vi "ITC503 Set Values.vi"(1 "Set Heater":dbl min=0.0 max=100.0 step=0.1 format="%.1f", 2 "Set Channel":i16 min=0 max=100 step=1, 3 "ITC503 Settings":T1={"ITC503 Set Setpoint"=0.0, "ITC503 Set Auto Heater"=TRUE, "ITC503 Set Auto PID"=TRUE, "P"=0.0, "I"=0.0, "D"=0.0} {"D" min=0.0 max=100.0 step=0.1 format="%.1f"; "I" min=0.0 max=100.0 step=0.1 format="%.1f"; "P" min=0.0 max=100.0 step=0.1 format="%.1f"; "ITC503 Set Setpoint" min=-273.0 max=300000.0 step=0.1 format="%.1f"}, 4 "ITC Setup":T2={"Description"="", "IO Info"={"Address"={"Com Port"=1, "ISOBUS Address"=1, "GPIB Address"=24, "Communication"=enum."ISOBUS"}, "Version"=enum."ITC503", "Ch 1 dec places"=1, "Ch 2 dec places"=1, "Ch 3 dec places"=1, "Ch1 Name"="", "Ch2 Name"="", "Ch3 Name"=""}}) -> ()   [LabVIEW 2010]
uses:
  drivers/Oxford ITC/ITCAPPS.LLB/ITCSetup.ctl
  drivers/Oxford ITC/ITCSUBS.LLB/ITCIO.ctl
  drivers/Oxford ITC/BUSGEN.LLB/OxfordAddress.ctl
  drivers/Oxford ITC/ITCSUBS.LLB/ITCVersion.ctl
  TypeDefs/ITC503 Settings.ctl
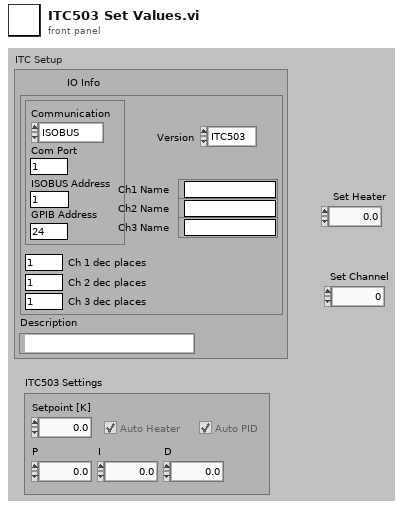
[diagram p1: front panel]
types:
  T1 = typedef "ITC503 Settings.ctl" = cluster{"ITC503 Set Setpoint":dbl, "ITC503 Set Auto Heater":bool, "ITC503 Set Auto PID":bool, "P":dbl, "I":dbl, "D":dbl}
  T2 = typedef "ITCSetup.ctl" = cluster{"Description":string, "IO Info":T3}
  T3 = typedef "ITCIO.ctl" = cluster{"Address":T4, "Version":T5, "Ch 1 dec places":i16, "Ch 2 dec places":i16, "Ch 3 dec places":i16, "Ch1 Name":string, "Ch2 Name":string, "Ch3 Name":string}
  T4 = typedef "OxfordAddress.ctl" = cluster{"Com Port":i32, "ISOBUS Address":i32, "GPIB Address":i16, "Communication":enum16{"RS232", "ISOBUS", "GPIB", "Gateway"}}
  T5 = typedef "ITCVersion.ctl" = enum16{"ITC502", "ITC503", "ITC601"}
  T6 = typedef "ITC503 Current Values.ctl" = cluster{"ITC503 Heater":dbl, "ITC503 Temperature":dbl, "ITC503 P":dbl, "ITC503 I":dbl, "ITC503 D":dbl, "ITC503 Setpoint":dbl, "ITC503 Gradient":dbl, "ITC503 Heater Auto":bool, "ITC503 PID Auto":bool}
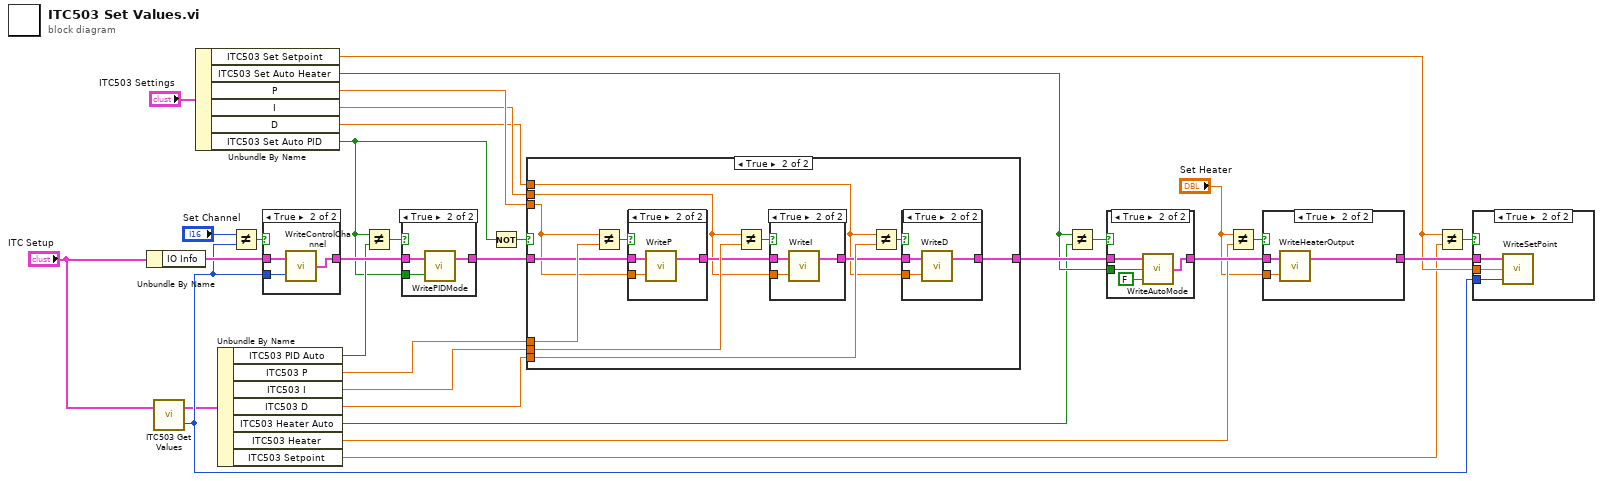
[diagram p0: block diagram]
diagram:
  n1 = Unbundle By Name("ITC Setup") -> ("IO Info"=w27:T3)
  n2 = call "ITC503 Get Values.vi"("ITC Setup"="ITC Setup") -> ("Control Channel"=w12:i16, "ITC503 Current Values"=w11:T6)  [unwired: 1 in]
  n3 = Unbundle By Name("ITC503 Settings") -> ("ITC503 Set Setpoint"=w13:dbl, "ITC503 Set Auto Heater"=w14:bool, "P"=w17:dbl, "I"=w16:dbl, "D"=w15:dbl, "ITC503 Set Auto PID"=w9:bool)
  n4 = Unbundle By Name(w11) -> ("ITC503 PID Auto"=w10:bool, "ITC503 P"=w8:dbl, "ITC503 I"=w6:dbl, "ITC503 D"=w7:dbl, "ITC503 Heater Auto"=w5:bool, "ITC503 Heater"=w4:dbl, "ITC503 Setpoint"=w3:dbl)
  n5 = Not Equal?(x="Set Channel", y=w12) -> (x != y?=w31:bool)
  n6 = case shown="True" w31 {
    tunnel: w27 -> [w32 w35]
    tunnel: w12 -> [_ w34]
    tunnel: [w32 w33] -> w26
    frame False {
    }
    frame True {
      n7 = call "WriteControlChannel.vi"("Control Channel"=w34, "ITC IO Info"=w35) -> ("ITC IO Info"=w33:T3)
    }
  }
  n8 = Not Equal?(x=w9, y=w10) -> (x != y?=w30:bool)
  n9 = case shown="True" w30 {
    tunnel: w26 -> [w36 w38]
    tunnel: w9 -> [_ w39]
    tunnel: [w36 w37] -> w23
    frame False {
    }
    frame True {
      n10 = call "WritePIDMode.vi"("Auto PID"=w39, "ITC IO Info"=w38) -> ("ITC IO Info"=w37:T3)  [unwired: 1 in]
    }
  }
  n11 = Not(x=w9) -> (.not. x?=w24:bool)
  n12 = case shown="True" w24 {
    tunnel: w8 -> [_ w50]
    tunnel: w7 -> [_ w49]
    tunnel: w6 -> [_ w48]
    tunnel: w23 -> [w40 w47]
    tunnel: [w40 w44] -> w22
    tunnel: w17 -> [_ w43]
    tunnel: w16 -> [_ w42]
    tunnel: w15 -> [_ w41]
    frame False {
    }
    frame True {
      n13 = Not Equal?(x=w43, y=w50) -> (x != y?=w51:bool)
      n14 = case shown="True" w51 {
        tunnel: w43 -> [_ w57]
        tunnel: w47 -> [w54 w56]
        tunnel: [w54 w55] -> w46
        frame False {
        }
        frame True {
          n15 = call "WriteP.vi"("P (% of span)"=w57, "ITC IO Info"=w56) -> ("ITC IO Info"=w55:T3)  [unwired: 1 in]
        }
      }
      n16 = Not Equal?(x=w42, y=w48) -> (x != y?=w53:bool)
      n17 = case shown="True" w53 {
        tunnel: w42 -> [_ w61]
        tunnel: w46 -> [w58 w60]
        tunnel: [w58 w59] -> w45
        frame False {
        }
        frame True {
          n18 = call "WriteI.vi"("I"=w61, "ITC IO Info"=w60) -> ("ITC IO Info"=w59:T3)  [unwired: 1 in]
        }
      }
      n19 = Not Equal?(x=w41, y=w49) -> (x != y?=w52:bool)
      n20 = case shown="True" w52 {
        tunnel: w41 -> [_ w65]
        tunnel: w45 -> [w62 w64]
        tunnel: [w62 w63] -> w44
        frame False {
        }
        frame True {
          n21 = call "WriteD.vi"("D"=w65, "ITC IO Info"=w64) -> ("ITC IO Info"=w63:T3)  [unwired: 1 in]
        }
      }
    }
  }
  n22 = Not Equal?(x=w14, y=w5) -> (x != y?=w29:bool)
  n23 = case shown="True" w29 {
    tunnel: w22 -> [w66 w70]
    tunnel: w14 -> [_ w69]
    tunnel: [w66 w68] -> w21
    frame False {
    }
    frame True {
      n24 = call "WriteAutoMode.vi"("Auto Needle Valve"=FALSE, "Auto Heat"=w69, "ITC IO Info"=w70) -> ("ITC IO Info"=w68:T3)
    }
  }
  n25 = Not Equal?(x="Set Heater", y=w4) -> (x != y?=w19:bool)
  n26 = case shown="True" w19 {
    tunnel: "Set Heater" -> [_ w74]
    tunnel: w21 -> [w71 w73]
    tunnel: [w71 w72] -> w20
    frame False {
    }
    frame True {
      n27 = call "WriteHeaterOutput.vi"("Heater Output (%)"=w74, "ITC IO Info"=w73) -> ("ITC IO Info"=w72:T3)  [unwired: 1 in]
    }
  }
  n28 = Not Equal?(x=w13, y=w3) -> (x != y?=w25:bool)
  n29 = case shown="True" w25 {
    tunnel: w20 -> [_ w77]
    tunnel: w13 -> [_ w76]
    tunnel: w12 -> [_ w75]
    frame False {
    }
    frame True {
      n30 = call "WriteSetPoint.vi"("Control Ch"=w75, "Set point"=w76, "IO Info"=w77) -> ()  [unwired: 1 out]
    }
  }
